vi "Builder.vi"(8 "error in (no error)":errorcluster, 11 "Config File Path":path) -> (0 "error out":errorcluster, 2 "return type":i32, 3 "Server out":refnum<class "Server.lvclass">)   [LabVIEW 2017, in "opcua.lvlib" / "Server.lvclass"]
uses:
  Server.lvclass
  Server.lvclass/Server.ctl
  opcua32.dll
  opcua.lvlib
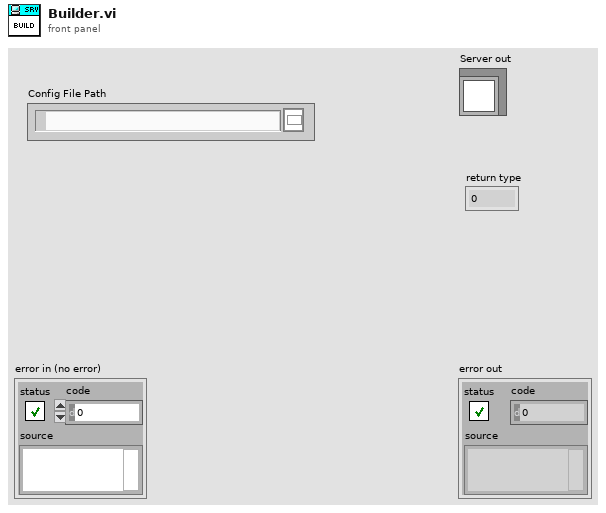
[diagram p1: front panel]
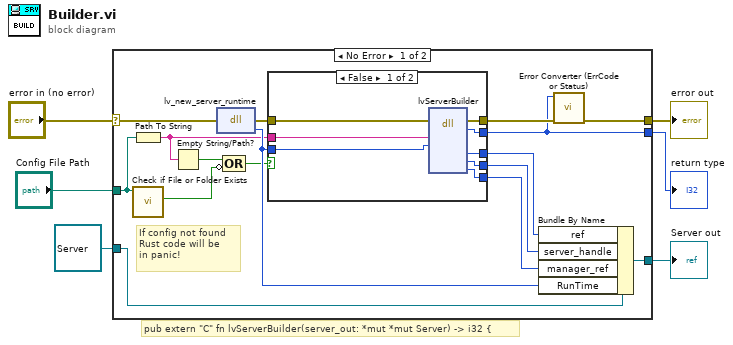
[diagram p0: block diagram]
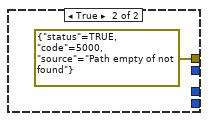
[diagram p2: hidden frame]
diagram:
  # "pub extern \"C\" fn lvServerBuilder(server_out: *mut *mut Server) -> i32 {"
  n1 = case shown="No Error" "error in (no error)" {
    selector: "error in (no error)" -> [w15 w32]
    tunnel: [w8 w32] -> w5
    tunnel: [w21 w33] -> w3
    tunnel: refnum<class "Server.lvclass"> refnum ("Server in") -> [w22 w33]
    tunnel: [w7 _] -> w2
    tunnel: "Config File Path" -> [w13 _]
    frame No Error {
      # "If config not found\nRust code will be\nin panic!"
      n2 = Path To String(path=w13) -> (string=w14:string)
      n3 = call <vilib>:"Check if File or Folder Exists.vi"("path"=w13) -> ("file or folder exists?"=w11:bool)  [unwired: 8 in, 2 out]
      n4 = Empty String/Path?(string/path=w14) -> (empty?=w12:bool)
      n5 = dll-call lib="C:/Users/Andrey/Desktop/opcua-labview/opcua-lvlib/opcua*.dll" fn="lv_new_server_runtime"(error in=w15) -> (error out=w20:errorcluster, "return type"=w16:u64)  [unwired: 2 in, 1 out]
      n6 = Compound Arithmetic op=OR(w12, invert w11) -> (w10:bool)
      n7 = case shown="False" w10 {
        tunnel: w20 -> [w30 _]
        tunnel: [w29 _] -> w19
        tunnel: [w28 _] -> w7
        tunnel: [w27 _] -> w18
        tunnel: [w26 _] -> w17
        tunnel: w16 -> [w25 _]
        tunnel: [w24 errorcluster {"status"=TRUE, "code"=5000, "source"="Path empty of not found"} ("error out")] -> w9
        tunnel: w14 -> [w23 _]
        frame False {
          n8 = dll-call lib="C:/Users/Andrey/Desktop/opcua-labview/opcua-lvlib/opcua*.dll" fn="lvServerBuilder"(error in=w30, "config_path"=w23, "runtime"=w25) -> (error out=w24:errorcluster, "return type"=w28:i32, "server_ref"=w29:u64, "server_handle"=w27:u64, "server_manager"=w26:u64)  [unwired: 7 in, 1 out]
        }
        frame True {
        }
      }
      n9 = Bundle By Name(cluster=w22, "ref"=w19, "server_handle"=w18, "manager_ref"=w17, "RunTime"=w16) -> (w21:refnum<class "Server.lvclass">)
      n10 = call "Error Converter (ErrCode or Status).vi"("error in (no error)"=w9, "error code"=w7) -> ("error out"=w8:errorcluster)  [unwired: 9 in]
    }
    frame Error {
    }
  }
  "error out" <- w5
  "Server out" <- w3
  "return type" <- w2
